vi "sub_udp_main_master.vi"(8 "error in":errorcluster) -> (0 "error out":errorcluster)   [LabVIEW 2019]
uses:
  Ctrl/cmd_common.ctl
panel:
  out "receive":string
  out "n":i32
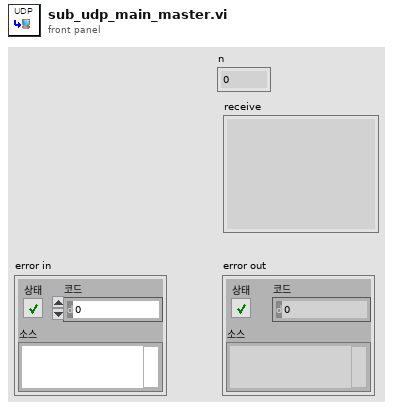
[diagram p1: front panel]
types:
  T1 = typedef "cmd_common.ctl" = enum16{"read", "write"}
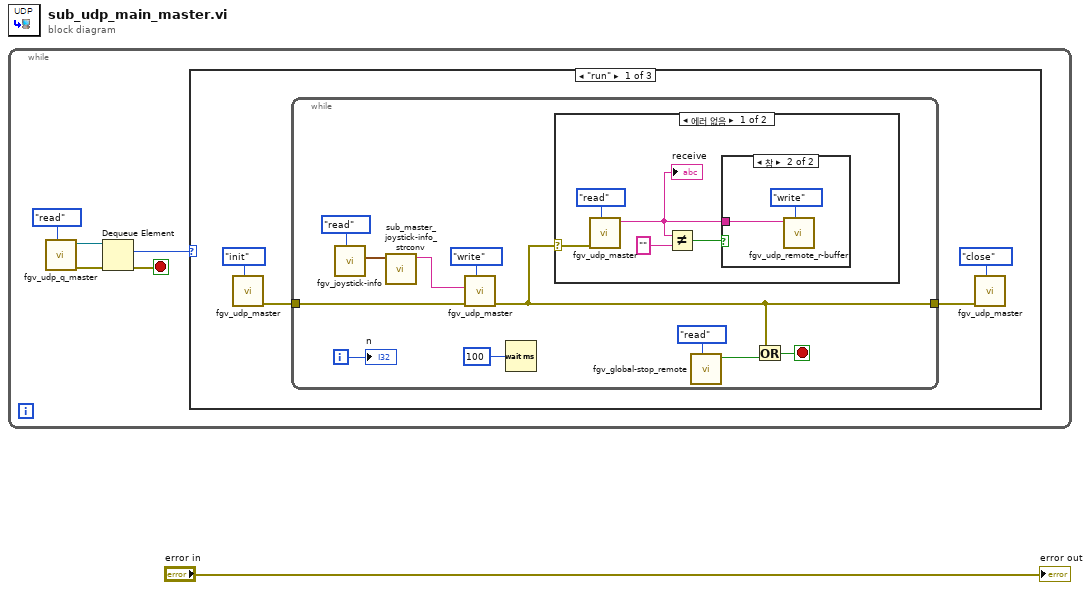
[diagram p0: block diagram]
diagram:
  n1 = while {
    stop <- w2 stop-if-true
    n2 = call "fgv_udp_q_master.vi"("cmd"=enum16{"create", "write", "read", "close"}."read") -> ("error out"=w4:errorcluster, "queue out"=w5:refnum<queue>)  [unwired: 9 in]
    n3 = Dequeue Element(queue=w5, error in (no error)=w4) -> (element=w3:enum16{"run", "check", "stop"}, error out=w2:errorcluster)  [unwired: 1 in, 2 out]
    n4 = case shown="\"run\"" w3 {
      frame "run" {
        n5 = call "fgv_udp_master.vi"("cmd"=enum16{"init", "read", "write", "close"}."init") -> ("error out"=w9:errorcluster)  [unwired: 9 in, 1 out]
        n6 = while {
          tunnel: w9 -> [w20]
          tunnel: [w14] -> w10
          i -> [w15]
          stop <- w19 stop-if-true
          n7 = call "fgv_joystick-info.vi"("init"=enum16{"enable", "init", "read", "write"}."read") -> ("v_val"=w18:cluster{dbl, dbl})  [unwired: 7 in, 3 out]
          n8 = call "sub_master_joystick-info_strconv.vi"("velocity"=w18) -> ("str out"=w17:string)  [unwired: 10 in]
          n9 = call "fgv_udp_master.vi"("cmd"=enum16{"init", "read", "write", "close"}."write", "error in"=w20, "send data"=w17) -> ("error out"=w14:errorcluster)  [unwired: 7 in, 1 out]
          n10 = Wait (ms)(milliseconds to wait=u32 100 ("dt")) -> ()  [unwired: 1 out]
          n11 = case shown="에러 없음" w14 {
            selector: w14 -> [w25 _]
            frame No Error {
              n12 = call "fgv_udp_master.vi"("cmd"=enum16{"init", "read", "write", "close"}."read", "error in"=w25) -> ("receive"=w23:string)  [unwired: 8 in, 1 out]
              "receive" <- w23
              n13 = Not Equal?(x=w23, y="") -> (x != y?=w24:bool)
              n14 = case shown="참" w24 {
                tunnel: w23 -> [_ w27]
                frame False {
                }
                frame True {
                  n15 = call "fgv_udp_remote_r-buffer.vi"("cmd"=cmd_common."write", "udp r buff"=w27) -> ()  [unwired: 9 in, 1 out]
                }
              }
            }
            frame Error {
            }
          }
          n16 = call "fgv_global-stop_remote.vi"("cmd"=enum16{"ini", "read", "stop"}."read") -> ("stop status"=w12:bool)  [unwired: 10 in]
          n17 = Or(x=w14, y=w12) -> (x .or. y?=w19:bool)
          "n" <- w15
        }
        n18 = call "fgv_udp_master.vi"("cmd"=enum16{"init", "read", "write", "close"}."close", "error in"=w10) -> ()  [unwired: 8 in, 2 out]
      }
      frame "check" {
      }
      frame "stop", Default {
      }
    }
  }
  "error out" <- "error in"
